vi "Transfer Configuration.Required Buffer Size.vi"(8 "error in (no error)":errorcluster, 11 "Transfer Configuration in":refnum<class "Transfer Configuration.lvclass">) -> (0 "error out":errorcluster, 2 "required buffer size":u64 format="%d bytes", 3 "Transfer Configuration out":refnum<class "Transfer Configuration.lvclass">)   [LabVIEW 2017, in "DSF Core.lvlib" / "Transfer Configuration.lvclass"]
uses:
  Transfer Configuration.lvclass
  Transfer Configuration.lvclass/Transfer Configuration.ctl
  VIs/DSF.Data Type.Sizeof.vi
  DSF Core.lvlib
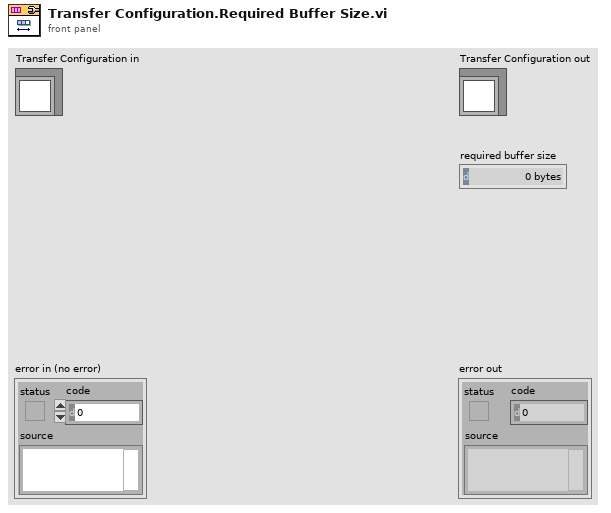
[diagram p1: front panel]
types:
  T1 = typedef "DSF Core.lvlib/DSF Runtime Channel Block.ctl" = cluster{"data type":T2, "count":u64, "buffer offset":u64}
  T2 = typedef "DSF Core.lvlib/DSF Data Type.ctl" = enum8{"Bool", "SGL", "DBL", "I8", "I16", "I32", "I64", "U8", "U16", "U32", "U64"}
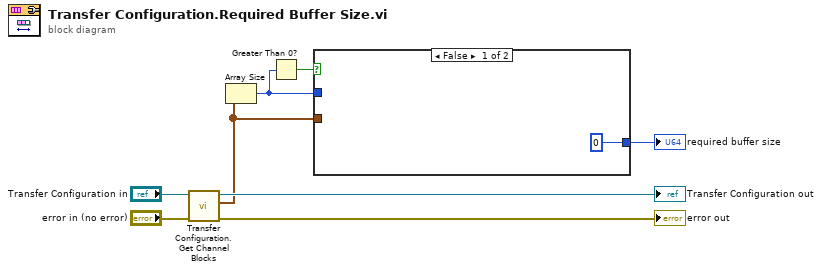
[diagram p0: block diagram]
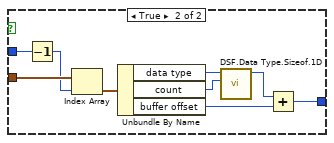
[diagram p2: hidden frame]
diagram:
  n1 = call "Transfer Configuration.Get Channel Blocks.vi"("Transfer Configuration in"="Transfer Configuration in") -> ("channel blocks"=w2:T1[], "Transfer Configuration out"=→"Transfer Configuration out":refnum<class "Transfer Configuration.lvclass">)  [unwired: 9 in]
  n2 = Array Size(array=w2) -> (size(s)=w4:i32)
  n3 = Greater Than 0?(x=w4) -> (x > 0?=w3:bool)
  n4 = case shown="False" w3 {
    tunnel: w4 -> [_ w17]
    tunnel: w2 -> [_ w16]
    tunnel: [u64 0 w9] -> w1
    frame False {
    }
    frame True {
      n5 = Decrement(x=w17) -> (x-1=w15:i32)
      n6 = Index Array(array=w16, index=w15) -> (element=w14:T1)
      n7 = Unbundle By Name(w14) -> ("data type"=w13:T2, "count"=w12:u64, "buffer offset"=w11:u64)
      n8 = call "DSF.Data Type.Sizeof.1D.vi"("count"=w12, "data type"=w13) -> ("size in bytes"=w10:u64)  [unwired: 9 in]
      n9 = Add(x=w10, y=w11) -> (x+y=w9:u64)
    }
  }
  "required buffer size" <- w1
  "error out" <- "error in (no error)"
